vi "GUI_Single Button Pump.vi"() -> ()   [LabVIEW 2011]
uses:
  LB Status Named_typdef.ctl
  LB Statusboolarray1_typdef.ctl
  LB Statusboolarray2_typdef.ctl
  LB Statusboolarray3_typdef.ctl
  LB statusintegerarray_typdef.ctl
  LB statusfloatrarray_typdef.ctl
  EC Status Named_typdef.ctl
  EC Statusboolarray2_typdef.ctl
  EC Statusboolarray3_typdef.ctl
  EC Statusboolarray1_typdef.ctl
  EC statusintegerarray_typdef.ctl
  EC statusfloatrarray_typdef.ctl
  GPM Mode_typdef.ctl
  User Event Data Type typdef.ctl
  Error Action.ctl
  Error codes.ctl
  DecisionCluster_typdef.ctl
  MainCluster_typdef.ctl
  Chamber Selection_typdef.ctl
  timerAction_typdef.ctl
  action_typdef.ctl
  op_typdef.ctl
  Selection Action_typdef.ctl
  command_typdef.ctl
panel:
  in  "Tab Control":enum32{"Control", "Debug LB", "Debug EC"}(tab)
  in  "Pump":bool
  in  "Current State":string
  in  "Display Message":string
  in  "Errors/Warnings":i32(listbox)=1
  in  "OK":bool
  in  "GPM Mode":T1
  in  "Debug Mode?":bool
  in  "LB Status Named":T2
  in  "EC Status Named":T8
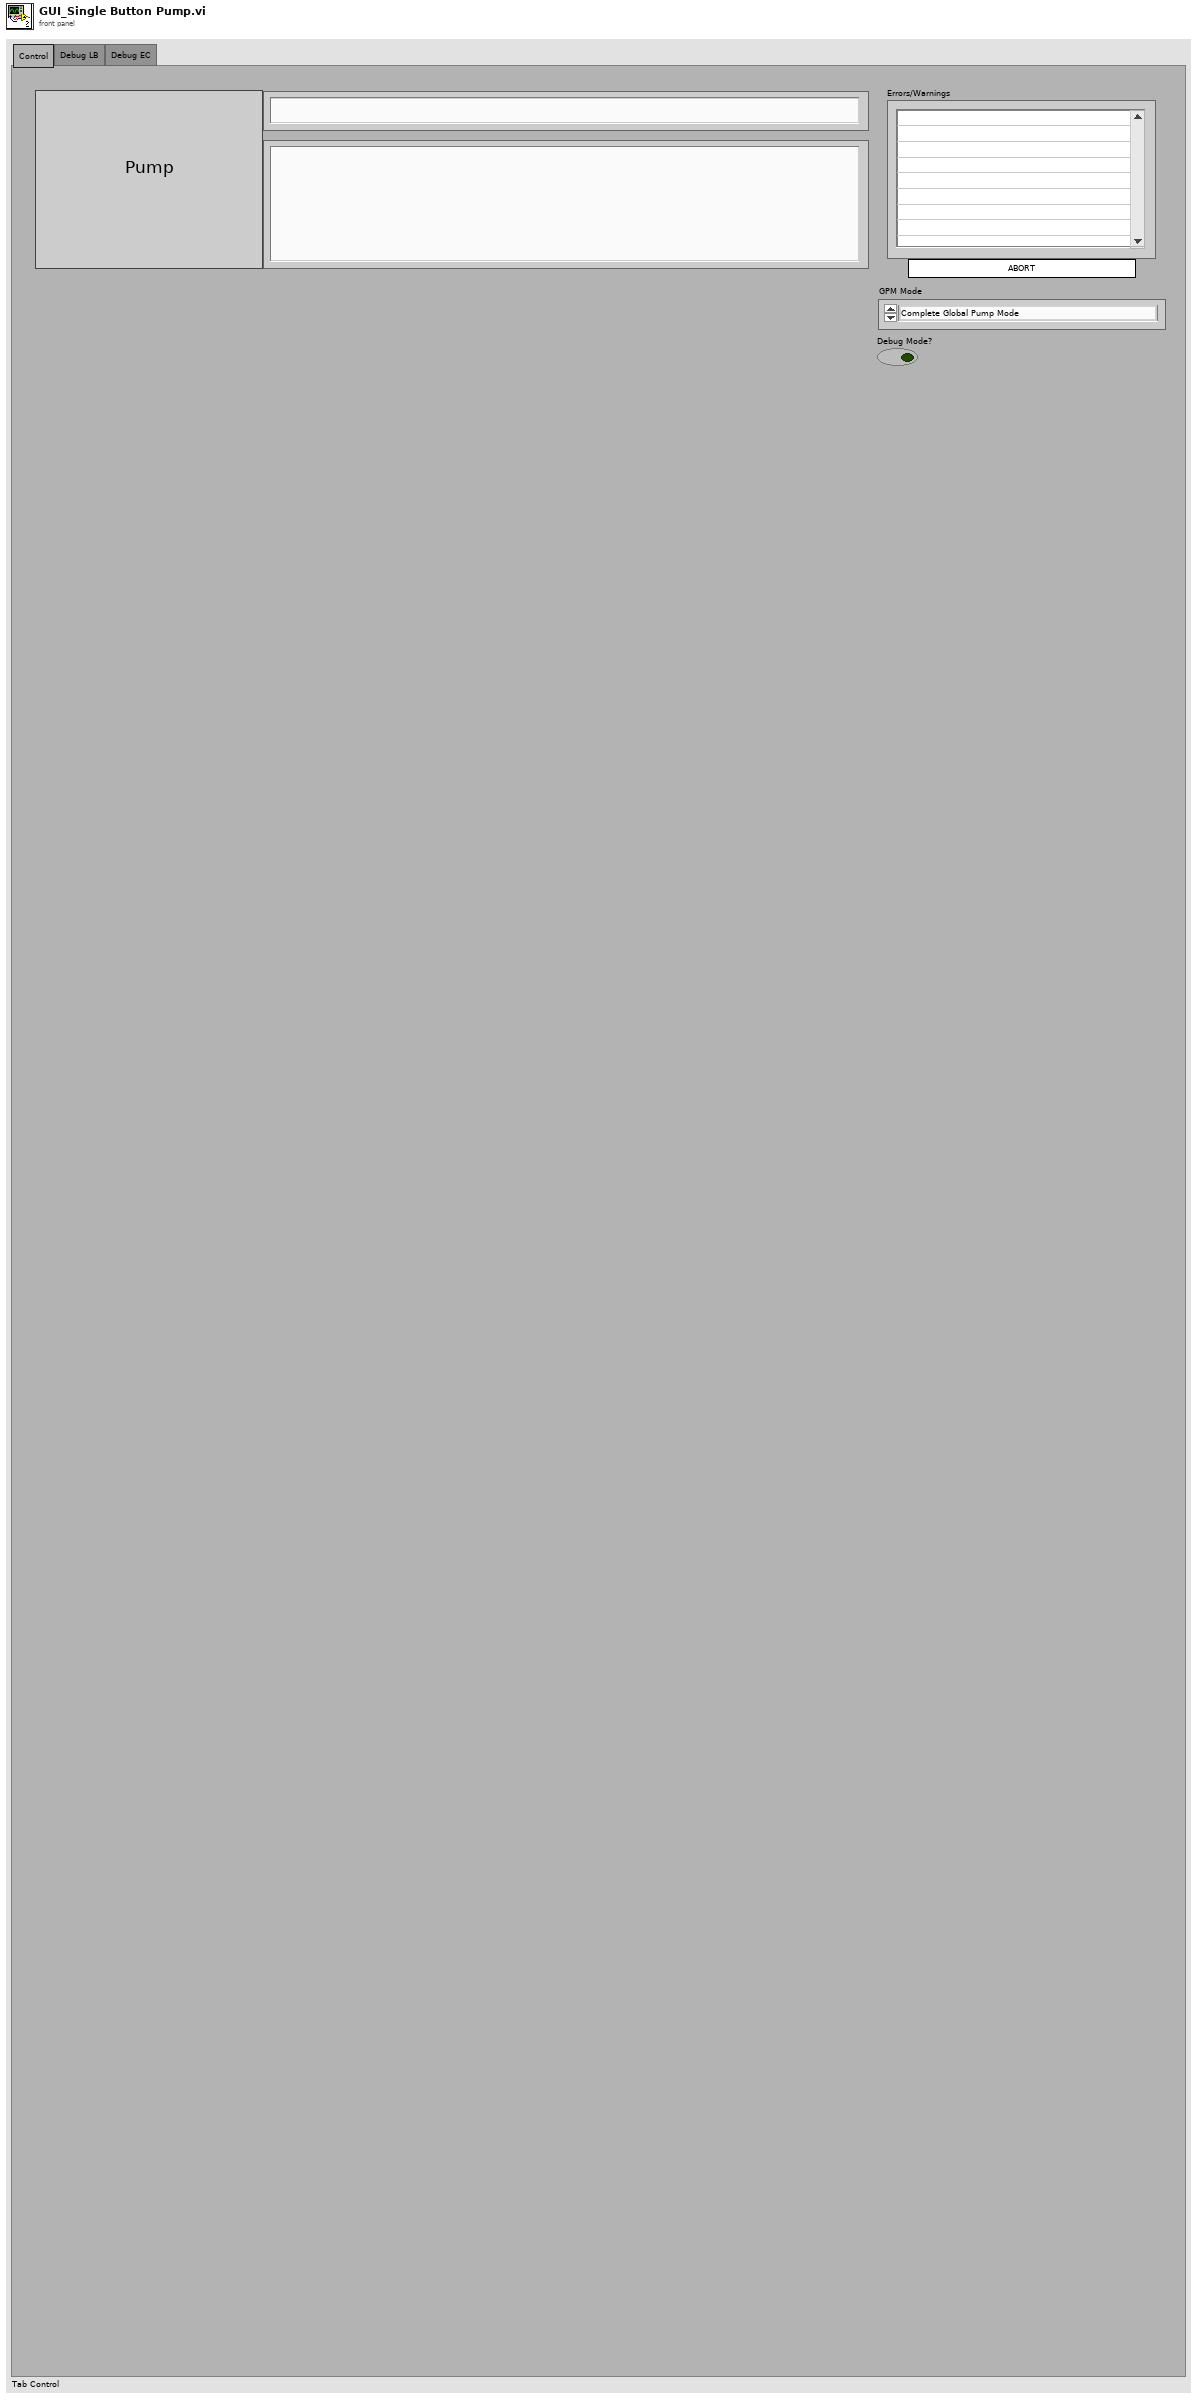
[diagram p1: front panel]
types:
  T1 = typedef "GPM Mode_typdef.ctl" = enum16{"Complete Global Pump Mode", "Selected Global Pump Mode"}
  T2 = typedef "LB Status Named_typdef.ctl" = cluster{"LB statusboolarray1":T3, "LB statusboolarray2":T4, "LB statusboolarray3":T5, "LB statusintegerarray":T6, "LB statusfloatarray":T7}
  T3 = typedef "LB Statusboolarray1_typdef.ctl" = cluster{"COMP ion gauge on feedback":bool, "COMP ion gauge degas feedback":bool, "M123 ion gauge on feedback":bool, "M123 ion gauge degas feedback":bool, "OAP ion gauge on feedback":bool, "OAP ion gauge degas feedback":bool, "Spare 1":bool, "Spare 2":bool, "Spare 3":bool, "Spare 4":bool, "Spare 5":bool, "Spare 6":bool, "ROUGHING MANIFOLD VALVE opened":bool, "ROUGHING MANIFOLD VALVE closed":bool, "BACKING MANIFOLD VALVE opened":bool, "BACKING MANIFOLD VALVE closed":bool, "ROUGHING BACKING CONNECT VALVE opened":bool, "ROUGHING BACKING CONNECT VALVE closed":bool, "COMPRESSOR ROUGHING VALVE opened":bool, "COMPRESSOR ROUGHING VALVE closed":bool, "M123 ROUGHING VALVE opened":bool, "M123 ROUGHING VALVE closed":bool, "BEAMDUMP ROUGHING VALVE opened":bool, "BEAMDUMP ROUGHING VALVE closed":bool, "OAP ROUGHING VALVE opened":bool, "OAP ROUGHING VALVE closed":bool, "GATE VALVE COMP-M123 opened":bool, "GATE VALVE COMP-M123 closed":bool, "GATE VALVE BEAM DUMP opened":bool, "GATE VALVE BEAM DUMP closed":bool, "GATE VALVE M123-OAP opened":bool, "GATE VALVE M123-OAP closed":bool, "GATE VALVE OAP-BTL opened":bool, "GATE VALVE OAP-BTL closed":bool, "COMPRESSOR VENT VALVE opened":bool, "COMPRESSOR VENT VALVE closed":bool, "M123 VENT VALVE opened":bool, "M123 VENT VALVE closed":bool, "BEAMDUMP VENT VALVE opened":bool, "BEAMDUMP VENT VALVE closed":bool, "OAP VENT VALVE opened":bool, "OAP VENT VALVE closed":bool, "COMPRESSOR Turbo Gate Valve opened ":bool, "COMPRESSOR Turbo Gate Valve closed":bool, "M123 Turbo Gate Valve opened":bool, "M123 Turbo Gate Valve closed":bool, "OAP Turbo Gate Valve opened":bool, "OAP Turbo Gate Valve closed":bool, "COMPRESSOR Turbo Backing Valve opened":bool, "COMPRESSOR Turbo Backing Valve closed":bool, "M123 Turbo Backing Valve opened":bool, "M123 Turbo Backing Valve closed":bool, "OAP Turbo Backing Valve opened":bool, "OAP Turbo Backing Valve closed":bool, "Roughing Manifold Vent Valve opened":bool, "Roughing Manifold Vent Valve closed":bool, "Spare 7":bool, "Spare 8":bool, "Spare 9":bool, "Spare 10":bool, "RP RUN opened":bool, "RP no FAULT closed":bool, "BP RUN opened":bool, "BP no FAULT closed":bool}
  T4 = typedef "LB Statusboolarray2_typdef.ctl" = cluster{"Spare 1":bool, "Spare 2":bool, "Spare 3":bool, "Spare 4":bool, "ROUGHING PUMP run":bool, "ROUGHING PUMP no fault":bool, "BACKING PUMP run":bool, "BACKING PUMP no fault":bool, "COMP TURBO fault feedback":bool, "COMP TURBO normal feedback":bool, "M123 TURBO fault feedback":bool, "M123 TURBO normal feedback":bool, "OAP TURBO fault feedback":bool, "OAP TURBO normal feedback":bool, "Spare 9":bool, "Spare 10":bool, "Spare 11":bool, "Spare 12":bool, "Spare 13":bool, "Spare 14":bool, "ROUGHING PUMP FLOW SWITCH":bool, "BACKING PUMP FLOW SWITCH":bool, "COMP TURBO FLOW SWITCH":bool, "M123 TURBO FLOW SWITCH":bool, "OAP TURBO FLOW SWITCH":bool, "Spare 15":bool, "Spare 16":bool, "Spare 17":bool, "COMP ion gauge on signal":bool, "COMP ion gauge degas signal":bool, "M123 ion gauge on signal":bool, "M123 ion gauge degas signal":bool, "OAP ion gauge on signal":bool, "OAP ion gauge degas signal":bool, "Spare 18":bool, "Spare 19":bool, "Spare 20":bool, "Spare 21":bool, "Spare 22":bool, "Spare 23":bool, "ROUGHING MANIFOLD VALVE":bool, "BACKING MANIFOLD VALVE":bool, "ROUGHING BACKING CONNECT VALVE":bool, "COMPRESSOR ROUGHING VALVE":bool, "M123 ROUGHING VALVE":bool, "BEAMDUMP ROUGHING VALVE":bool, "OAP ROUGHING VALVE":bool, "GATE VALVE COMP-M123":bool, "GATE VALVE BEAM DUMP":bool, "GATE VALVE M123-OAP":bool, "GATE VALVE OAP-BTL":bool, "COMPRESSOR VENT VALVE":bool, "M123 VENT VALVE":bool, "BEAMDUMP VENT VALVE":bool, "OAP VENT VALVE":bool, "COMPRESSOR Turbo Gate Valve":bool, "M123 Turbo Gate Valve":bool, "OAP Turbo Gate Valve":bool, "COMPRESSOR Turbo Backing Valve":bool, "M123 Turbo Backing Valve":bool, "OAP Turbo Backing Valve":bool, "Spare 24":bool, "Spare 25":bool, "Spare 26":bool}
  T5 = typedef "LB Statusboolarray3_typdef.ctl" = cluster{"Spare 1":bool, "Spare 2":bool, "Spare 3":bool, "Spare 4":bool, "ROUGHING PUMP":bool, "BACKING PUMP":bool, "Spare 5":bool, "Spare 6":bool, "Spare 7":bool, "Spare 8":bool, "Spare 9":bool, "COMP Turbo Vent Valve":bool, "M123 Turbo Vent Valve":bool, "OAP Turbo Vent Valve":bool, "Spare 10":bool, "Spare 11":bool, "Spare 12":bool, "Spare 13":bool, "COMP turbo pump run signal":bool, "M123 turbo pump run signal":bool, "OAP turbo pump run signal":bool, "Spare 14":bool, "Spare 15":bool, "Spare 16":bool, "watch dog timer - out":bool, "GATE OAP-BTL - closed out":bool, "GATE 1 – closed out":bool, "GATE 2 – closed out":bool, "GATE 3,4 – closed out":bool, "GPM LB - out":bool, "GVM LB - out":bool, "RP LB status - out":bool, "RP EC - toggle - out":bool, "Spare 17":bool, "Spare 18":bool, "Spare 19":bool, "Spare 20":bool, "Spare 21":bool, "Spare 22":bool, "Spare 23":bool}
  T6 = typedef "LB statusintegerarray_typdef.ctl" = cluster{"COMP vacuum status word convectron ATM":i32, "M123 vacuum status word convectron ATM":i32, "OAP vacuum status word convectron ATM":i32, "HPBD vacuum status word convectron ATM":i32, "Spare 1":i32, "Spare 2":i32, "roughing pump vacuum status word convectron":i32, "backing pump vacuum status word convectron":i32, "roughing manifold vacuum status word convectron":i32, "backing manifold vacuum status word convectron":i32, "COMP Convectron vacuum status word convectron":i32, "M123 Convectron vacuum status word convectron":i32, "OAP Convectron vacuum status word convectron":i32, "Spare 3":i32, "Spare 4":i32, "COMP status word turbo pump":i32, "M123 status word turbo pump":i32, "OAP status word turbo pump":i32, "Spare 5":i32, "Spare 6":i32, "Spare 7":i32, "Spare 8":i32, "Spare 9":i32, "Spare 10":i32, "COMP CONVECTRON consloidate":i32, "Spare 11":i32, "Spare 12":i32, "Spare 13":i32, "M123 CONVECTRON consloidate":i32, "Spare 14":i32, "Spare 15":i32, "Spare 16":i32, "OAP CONVECTRON consloidate":i32, "Spare 17":i32, "Spare 18":i32, "Spare 19":i32, "HPBD CONVECTRON consloidate":i32, "Spare 20":i32, "Spare 21":i32, "Spare 22":i32, "Spare 23":i32, "Spare 24":i32, "Spare 25":i32, "Spare 26":i32, "Spare 27":i32, "Spare 28":i32, "Spare 29":i32, "Spare 30":i32}
  T7 = typedef "LB statusfloatrarray_typdef.ctl" = cluster{"COMP READING ION GAUGE":dbl, "M123 READING ION GAUGE":dbl, "OAP READING ION GAUGE":dbl, "Spare 1":i32, "Spare 2":i32, "Spare 3":i32, "Spare 4":i32, "Spare 5":i32, "roughing pump CONVECTRON GAUGE":dbl, "backing pump CONVECTRON GAUGE":dbl, "roughing manifold CONVECTRON GAUGE":dbl, "backing manifold CONVECTRON GAUGE":dbl, "COMP Convectron CONVECTRON GAUGE":dbl, "M123 Convectron CONVECTRON GAUGE":dbl, "OAP Convectron CONVECTRON GAUGE":dbl, "Spare 6":i32, "Spare 7":i32, "Spare 8":i32, "Spare 9":i32, "Spare 10":i32, "Spare 11":i32, "Spare 12":i32, "Spare 13":i32, "Spare 14":i32}
  T8 = typedef "EC Status Named_typdef.ctl" = cluster{"EC statusboolarray2":T9, "EC statusboolarray3":T10, "EC statusboolarray1":T11, "EC statusintegerarray":T12, "EC statusfloatarray":T13}
  T9 = typedef "EC Statusboolarray2_typdef.ctl" = cluster{"Spare 1":bool, "Spare 2":bool, "Spare 3":bool, "Spare 4":bool, "ROUGHING PUMP run opened":bool, "ROUGHING PUMP no fault closed":bool, "BACKING PUMP run opened":bool, "BACKING PUMP no fault closed":bool, "BTL TURBO turbo fault feedback":bool, "BTL TURBO turbo normal feedback":bool, "TARGET 1 TURBO turbo fault feedback":bool, "TARGET 1 TURBO turbo normal feedback":bool, "TARGET 2 TURBO turbo fault feedback":bool, "TARGET 2 TURBO turbo normal feedback":bool, "BTL2 TURBO turbo fault feedback":bool, "BTL2 TURBO turbo normal feedback":bool, "HPD TURBO turbo fault feedback":bool, "HPD TURBO turbo normal feedback":bool, "Spare 5":bool, "Spare 6":bool, "ROUGHING PUMP FLOW SWITCH":bool, "BACKING PUMP FLOW SWITCH":bool, "BTL TURBO FLOW SWITCH":bool, "TARGET 1 TURBO FLOW SWITCH":bool, "TARGET 2 TURBO FLOW SWITCH":bool, "BTL2 TURBO FLOW SWITCH":bool, "HPD TURBO FLOW SWITCH":bool, "Spare 7":bool, "BTL ion gauge on signal":bool, "BTL ion gauge degas signal":bool, "TARGET ion gauge on signal":bool, "TARGET ion gauge degas signal":bool, "BTL2 ion gauge on signal":bool, "BTL2 ion gauge degas signal":bool, "HPD ion gauge on signal":bool, "HPD ion gauge degas signal":bool, "Spare 8":bool, "Spare 9":bool, "Spare 10":bool, "Spare 11":bool, "ROUGHING MANIFOLD VALVE":bool, "BACKING MANIFOLD VALVE":bool, "ROUGHING BACKING CONNECT VALVE":bool, "BTL ROUGHING VALVE":bool, "BTL VENT VALVE":bool, "BTL Turbo Gate Valve":bool, "BTL Turbo Backing Valve":bool, "Roughing Manifold VV":bool, "Backing Manifold VV":bool, "TARGET ROUGHING VALVE":bool, "BTL2 ROUGHING VALVE":bool, "HPD ROUGHING VALVE":bool, "GV BTL-TARGET":bool, "GV TARGET-BTL2":bool, "GV BTL2-HPD":bool, "TARGET VENT VALVE":bool, "BTL2 VENT VALVE":bool, "HPD VENT VALVE":bool, "TARGET  Turbo Gate Valve 1":bool, "TARGET  Turbo Gate Valve 2":bool, "BTL2 Turbo Gate Valve":bool, "HPD  Turbo Gate Valve":bool, "TARGET Turbo Backing Valve 1":bool, "TARGET Turbo Backing Valve 2":bool}
  T10 = typedef "EC Statusboolarray3_typdef.ctl" = cluster{"BTL2 Turbo Backing Valve":bool, "HPD Turbo Backing Valve":bool, "Spare 1":bool, "Spare 2":bool, "Spare 3":bool, "Spare 4":bool, "Spare 5":bool, "Spare 6":bool, "Spare 7":bool, "Spare 8":bool, "Spare 9":bool, "BTL Turbo Vent Valve":bool, "TARGET1 Turbo Vent Valve":bool, "TARGET2 Turbo Vent Valve":bool, "BTL2 Turbo Vent Valve":bool, "HPD Turbo Vent Valve":bool, "Spare 10":bool, "Spare 11":bool, "BTL turbo pump run signal":bool, "TARGET1 turbo pump run signal":bool, "TARGET2 turbo pump run signal":bool, "BTL2 turbo pump run signal":bool, "HPD turbo pump run signal":bool, "Spare 12":bool, "watch dog timer - out":bool, "BTL vented – out":bool, "BTL medvac – out":bool, "BTL hivac – out":bool, "GPM EC - out":bool, "GVM EC - out":bool, "RP EC status - out":bool, "RP LB toggle - out":bool, "GATE ALL - closed out":bool, "Spare 13":bool, "Spare 14":bool, "Spare 15":bool, "Spare 16":bool, "Spare 17":bool, "Spare 18":bool, "Spare 19":bool, "Spare 20":bool, "Spare 21":bool, "Spare 22":bool, "Spare 23":bool, "Spare 24":bool, "Spare 25":bool, "Spare 26":bool, "Spare 27":bool}
  T11 = typedef "EC Statusboolarray1_typdef.ctl" = cluster{"BTL ion gauge on feedback":bool, "BTL ion gauge degas feedback":bool, "TARGET ion gauge on feedback":bool, "TARGET ion gauge degas feedback":bool, "BTL2 ion gauge on feedback":bool, "BTL2 ion gauge degas feedback":bool, "HPD ion gauge on feedback":bool, "HPD ion gauge degas feedback":bool, "Spare 1":bool, "Spare 2":bool, "Spare 3":bool, "Spare 4":bool, "ROUGHING MANIFOLD VALVE opened":bool, "ROUGHING MANIFOLD VALVE closed":bool, "BACKING MANIFOLD VALVE opened":bool, "BACKING MANIFOLD VALVE closed":bool, "ROUGHING BACKING CONNECT VALVE opened":bool, "ROUGHING BACKING CONNECT VALVE closed":bool, "BTL ROUGHING VALVE opened":bool, "BTL ROUGHING VALVE closed":bool, "BTL VENT VALVE opened":bool, "BTL VENT VALVE closed":bool, "BTL Turbo Gate Valve opened":bool, "BTL Turbo Gate Valve closed":bool, "BTL Turbo Backing Valve opened":bool, "BTL Turbo Backing Valve closed":bool, "Roughing Manifold VV opened":bool, "Roughing Manifold VV closed":bool, "Backing Manifold VV opened":bool, "Backing Manifold VV closed":bool, "TARGET ROUGHING VALVE opened":bool, "TARGET ROUGHING VALVE closed":bool, "BTL2 ROUGHING VALVE opened":bool, "BTL2 ROUGHING VALVE closed":bool, "HPD ROUGHING VALVE opened":bool, "HPD ROUGHING VALVE closed":bool, "GV BTL-TARGET opened":bool, "GV BTL-TARGET closed":bool, "GV TARGET-BTL2 opened":bool, "GV TARGET-BTL2 closed":bool, "GV BTL2-HPD opened":bool, "GV BTL2-HPD closed":bool, "TARGET VENT VALVE opened":bool, "TARGET VENT VALVE closed":bool, "BTL2 VENT VALVE opened":bool, "BTL2 VENT VALVE closed":bool, "HPD VENT VALVE opened":bool, "HPD VENT VALVE closed":bool, "TARGET  Turbo Gate Valve 1 opened":bool, "TARGET  Turbo Gate Valve 1 closed":bool, "TARGET  Turbo Gate Valve 2 opened":bool, "TARGET  Turbo Gate Valve 2 closed":bool, "BTL2 Turbo Gate Valve opened":bool, "BTL2 Turbo Gate Valve closed":bool, "HPD  Turbo Gate Valve opened":bool, "HPD  Turbo Gate Valve closed":bool, "TARGET Turbo Backing Valve 1 opened":bool, "TARGET Turbo Backing Valve 1 closed":bool, "TARGET Turbo Backing Valve 2 opened":bool, "TARGET Turbo Backing Valve 2 closed":bool, "BTL2 Turbo Backing Valve opened":bool, "BTL2 Turbo Backing Valve closed":bool, "HPD Turbo Backing Valve opened":bool, "HPD Turbo Backing Valve closed":bool}
  T12 = typedef "EC statusintegerarray_typdef.ctl" = cluster{"BTL vacuum status word convectron ATM":i32, "TARGET vacuum status word convectron ATM 2":i32, "BTL2 vacuum status word convectron ATM 3":i32, "HPD vacuum status word convectron ATM 4":i32, "Spare 1":i32, "Spare 2":i32, "roughing pump vacuum status word convectron":i32, "backing pump vacuum status word convectron":i32, "roughing manifold vacuum status word convectron":i32, "backing manifold vacuum status word convectron":i32, "BTL Convectron vacuum status word convectron":i32, "TARGET1 Convectron vacuum status word convectron":i32, "TARGET2 Convectron vacuum status word convectron":i32, "BTL2 Convectron vacuum status word convectron":i32, "HPD Convectron vacuum status word convectron":i32, "BTL status word turbo pump":i32, "TARGET1 status word turbo pump":i32, "TARGET2 status word turbo pump":i32, "BTL2 status word turbo pump??":i32, "HPD status word turbo pump":i32, "Spare 3":i32, "Spare 4":i32, "Spare 5":i32, "Spare 6":i32, "BTL CONVECTRON Consolidate":i32, "Spare 7":i32, "Spare 8":i32, "Spare 9":i32, "TARGET Consolidate":i32, "Spare 10":i32, "Spare 11":i32, "Spare 12":i32, "BTL2 Consolidate":i32, "Spare 13":i32, "Spare 14":i32, "Spare 15":i32, "HPD Consolidate":i32, "Spare 16":i32, "Spare 17":i32, "Spare 18":i32, "Spare 19":i32, "Spare 20":i32, "Spare 21":i32, "Spare 22":i32, "Spare 23":i32, "Spare 24":i32, "Spare 25":i32, "Spare 26":i32}
  T13 = typedef "EC statusfloatrarray_typdef.ctl" = cluster{"BTL READING ION GAUGE":dbl, "TARGET READING ION GAUGE":dbl, "BTL2 READING ION GAUGE":dbl, "HPD READING ION GAUGE":dbl, "Spare 1":dbl, "Spare 2":dbl, "Spare 3":dbl, "Spare 4":dbl, "roughing pump READING CONVECTRON GAUGE":dbl, "backing pump READING CONVECTRON GAUGE":dbl, "roughing manifold READING CONVECTRON GAUGE":dbl, "backing manifold READING CONVECTRON GAUGE":dbl, "BTL Convectron READING CONVECTRON GAUGE":dbl, "TARGET1 READING CONVECTRON GAUGE":dbl, "TARGET2 READING CONVECTRON GAUGE":dbl, "BTL2 READING CONVECTRON GAUGE":dbl, "HPD READING CONVECTRON GAUGE":dbl, "Spare 5":dbl, "Spare 6":dbl, "Spare 7":dbl, "Spare 8":dbl, "Spare 9":dbl, "Spare 10":dbl, "Spare 11":dbl}
  T14 = typedef "DecisionCluster_typdef.ctl" = cluster{"vi path":path, "Message":string}
  T15 = typedef "User Event Data Type typdef.ctl" = cluster{"Error Action":T16, "Error Codes":T17, "Status Array":string[]}
  T16 = typedef "Error Action.ctl" = enum16{"Add", "Remove", "Read All"}
  T17 = typedef "Error codes.ctl" = enum16{"001-GPM and GVM conditions", "002-Turbo gate valve status", "003-Chamber Gate Valve Status", "004-Check Chamber Pressures", "005-Check GPM Handshake", "006-Roughing Pump Status", "007-Backing Pump Status", "008-Backing valve status", "009-Roughing Manifold Pressure Status", "010-Roughing Valve Status", "011-Roughing Pump Status", "012-Turbo Backing Valve Status", "013-MID-VAC Status", "999-No Event"}
  T18 = enum8{"Enabled", "Disabled", "Disabled and Grayed Out"}
  T19 = enum32{"invalid app kind", "Development System", "Run Time System", "Student Edition", "Embedded LabVIEW", "Evaluation", "Custom"}
  T20 = typedef "MainCluster_typdef.ctl" = cluster{"Isolate HPBD":bool, "Core":cluster{"Current VI Reference":refnum<vi>, "Close Panel on Exit?":bool}, "Status Display Array":string[], "Connection URLs":cluster{"Source_URL EC":string, "Target_URL EC":string, "Source_URL LB":string, "Target_URL LB":string}, "EC Status":cluster{"bits 2":bool[], "bits 2":bool[], "bits 2":bool[], i32[], "FLOAT NUMBERS 2":sgl[]}, "EC Status Named":T8, "TCPConnection":cluster{"Status TCP Connection EC":refnum<k5>, "Command TCP Connection EC":refnum<k5>, "Status TCP Connection LB":refnum<k5>, "Command TCP Connection LB":refnum<k5>}, "EC Command Cluster":cluster{"boolarray1":cluster{bool, bool, bool, bool, bool, bool, bool, bool, bool, bool, bool, bool, bool, bool, bool, bool}, "boolarray2":cluster{bool, bool, bool, bool, bool, bool, bool, bool, bool, bool, bool, bool, bool, bool, bool, bool}, "boolarray3":cluster{bool, bool, bool, bool, bool, bool, bool, bool, bool, bool, bool, bool, bool, bool, bool, bool}, "boolarray4":cluster{bool, bool, bool, bool, bool, bool, bool, bool, bool, bool, bool, bool, bool, bool, bool, bool}}, "EC Command Named":cluster{"EC Command array 1":cluster{"ROUGHING MANIFOLD VALVE":bool, "BACKING MANIFOLD VALVE":bool, "ROUGHING BACKING CONNECT VALVE":bool, "BTL ROUGHING VALVE":bool, "BTL VENT VALVE":bool, "BTL Turbo Gate Valve":bool, "BTL Turbo Backing Valve":bool, "Roughing Manifold VV":bool, "Backing Manifold VV":bool, "TARGET ROUGHING VALVE":bool, "BTL2 ROUGHING VALVE":bool, "HPD ROUGHING VALVE":bool, "GV BTL-TARGET":bool, "GV TARGET-BTL2":bool, "GV BTL2-HPD":bool, "TARGET VENT VALVE":bool}, " EC Command array 2":cluster{"BTL2 VENT VALVE":bool, "HPD VENT VALVE":bool, "TARGET  Turbo Gate Valve 1":bool, "TARGET  Turbo Gate Valve 2":bool, "BTL2 Turbo Gate Valve":bool, "HPD  Turbo Gate Valve":bool, "TARGET Turbo Backing Valve 1":bool, "TARGET Turbo Backing Valve 2":bool, "BTL2 Turbo Backing Valve":bool, "HPD Turbo Backing Valve":bool, "Spare 1":bool, "Spare 2":bool, "ROUGHING PUMP":bool, "BACKING PUMP":bool, "Spare 3":bool, "Spare 4":bool}, "EC Command array 3":cluster{"Spare 1":bool, "Spare 2":bool, "Spare 3":bool, "BTL Turbo Vent Valve":bool, "TARGET1 Turbo Vent Valve":bool, "TARGET2 Turbo Vent Valve":bool, "BTL2 Turbo Vent Valve":bool, "HPD Turbo Vent Valve":bool, "Spare 4":bool, "Spare 5":bool, "GPM":bool, "GVM":bool, "Spare 6":bool, "BTL turbo pump":bool, "TARGET1 turbo pump":bool, "TARGET2 turbo pump":bool}, "EC Command array 4":cluster{"BLT turbo pump":bool, "HPD turbo pump":bool, "Spare 1":bool, "BTL ION GAUGE ion gauge":bool, "BTL ION GAUGE  ion gauge degas":bool, "TARGET ion gauge":bool, "TARGET ion gauge degas":bool, "BTL2 ion gauge":bool, "BTL2 ion gauge degas":bool, "HPD ion gauge":bool, "HPD ion gauge degas":bool, "Spare 2":bool, "Spare 3":bool, "Spare 4":bool, "Spare 5":bool, "Spare 6":bool}}, "LB Status Named":T2, "LB Status":cluster{"bits 2":bool[], "bits 2":bool[], "bits 2":bool[], i32[], "FLOAT NUMBERS 2":sgl[]}, "LB Command Cluster":cluster{"boolarray1":cluster{bool, bool, bool, bool, bool, bool, bool, bool, bool, bool, bool, bool, bool, bool, bool, bool}, "boolarray2":cluster{bool, bool, bool, bool, bool, bool, bool, bool, bool, bool, bool, bool, bool, bool, bool, bool}, "boolarray3":cluster{bool, bool, bool, bool, bool, bool, bool, bool, bool, bool, bool, bool, bool, bool, bool, bool}, "boolarray4":cluster{bool, bool, bool, bool, bool, bool, bool, bool, bool, bool, bool, bool, bool, bool, bool, bool}}, "LB Command Named":cluster{"LB commandarray1":cluster{"ROUGHING MANIFOLD VALVE":bool, "BACKING MANIFOLD VALVE":bool, "ROUGHING BACKING CONNECT VALVE":bool, "COMPRESSOR ROUGHING VALVE":bool, "M123 ROUGHING VALVE":bool, "BEAMDUMP ROUGHING VALVE":bool, "OAP ROUGHING VALVE":bool, "GATE VALVE COMP-M123":bool, "GATE VALVE BEAM DUMP":bool, "GATE VALVE M123-OAP":bool, "GATE VALVE OAP-BTL":bool, "COMPRESSOR VENT VALVE":bool, "M123 VENT VALVE":bool, "BEAMDUMP VENT VALVE":bool, "OAP VENT VALVE":bool, "COMPRESSOR Turbo Gate Valve":bool}, "LB commandarray2":cluster{"M123 Turbo Gate Valve":bool, "OAP Turbo Gate Valve":bool, "COMPRESSOR Turbo Backing Valve":bool, "M123 Turbo Backing Valve":bool, "OAP Turbo Backing Valve":bool, "Roughing Manifold Vent Valve":bool, "Backing Manifold Vent Valve":bool, "Spare 1":bool, "Spare 2":bool, "Spare 3":bool, "Spare 4":bool, "Spare 5":bool, "ROUGHING PUMP":bool, "BACKING PUMP":bool, "Spare 6":bool, "Spare 7":bool}, "LB commandarray3":cluster{"Spare 1":bool, "Spare 2":bool, "Spare 3":bool, "COMP Turbo Vent Valve":bool, "M123 Turbo Vent Valve":bool, "OAP Turbo Vent Valve":bool, "Spare 4":bool, "Spare 5":bool, "Spare 6":bool, "Spare 7":bool, "GPM":bool, "GVM":bool, "Spare 8":bool, "COMP turbo pump":bool, "M123 turbo pump":bool, "OAP turbo pump":bool}, "LB commandarray4":cluster{"Spare 1":bool, "Spare 2":bool, "Spare 3":bool, "COMP ION GAUGE":bool, "COMP ION GAUGE degas":bool, "M123 ION GAUGE":bool, "M123 ION GAUGE degas":bool, "OAP ION GAUGE":bool, "OAP ION GAUGE degas":bool, "Spare 4":bool, "Spare 5":bool, "Spare 6":bool, "Spare 7":bool, "Spare 8":bool, "Spare 9":bool, "Spare 10":bool}}, "VI Refnum":refnum<vi>, "Chamber Selection":T21, "GPM Mode":T1, "Debug Mode?":bool, "State Sanity Check Array":bool[], "Critical Failures":cluster{"GPM Exit?":bool}, "Comm Ready?":bool, "Status Reconnect Attempt":dbl}
  T21 = typedef "Chamber Selection_typdef.ctl" = cluster{"COMP":bool, "M123":bool, "HPBD":bool, "OAP":bool, "BTL":bool, "TARGET":bool, "BTL2":bool, "HPD":bool}
  T22 = typedef "timerAction_typdef.ctl" = enum16{"Idle", "Start Timer", "Timer Running"}
  T23 = enum32{"Invalid", "Standard", "Closed", "Hidden", "Minimized", "Maximized"}
  T24 = typedef "op_typdef.ctl" = enum16{"Idle", "Continue to Wait", "Exit", "Ignore and Continue"}
  T25 = typedef "Selection Action_typdef.ctl" = enum16{"No Action", "Check Chamber Pressure", "Check Turbo Gate Valves", "Open Turbo Backing Valves", "Check Turbo Backing Valves", "Check MID-VAC on Chambers", "Start Turbo Pumps", "Check Turbo Normal Operation", "Check Chamber Pressures", "Roughing Valve Selection"}
  T26 = cluster{"bits 2":bool[], "bits 2":bool[], "bits 2":bool[], i32[], "FLOAT NUMBERS 2":sgl[]}
  T27 = cluster{"bits 2[0]":bool, "bits 2[1]":bool, "bits 2[2]":bool, "bits 2[3]":bool, "bits 2[4]":bool, "bits 2[5]":bool, "bits 2[6]":bool, "bits 2[7]":bool, "bits 2[8]":bool, "bits 2[9]":bool, "bits 2[10]":bool, "bits 2[11]":bool, "bits 2[12]":bool, "bits 2[13]":bool, "bits 2[14]":bool, "bits 2[15]":bool, "bits 2[16]":bool, "bits 2[17]":bool, "bits 2[18]":bool, "bits 2[19]":bool, "bits 2[20]":bool, "bits 2[21]":bool, "bits 2[22]":bool, "bits 2[23]":bool, "bits 2[24]":bool, "bits 2[25]":bool, "bits 2[26]":bool, "bits 2[27]":bool, "bits 2[28]":bool, "bits 2[29]":bool, "bits 2[30]":bool, "bits 2[31]":bool, "bits 2[32]":bool, "bits 2[33]":bool, "bits 2[34]":bool, "bits 2[35]":bool, "bits 2[36]":bool, "bits 2[37]":bool, "bits 2[38]":bool, "bits 2[39]":bool, "bits 2[40]":bool, "bits 2[41]":bool, "bits 2[42]":bool, "bits 2[43]":bool, "bits 2[44]":bool, "bits 2[45]":bool, "bits 2[46]":bool, "bits 2[47]":bool, "bits 2[48]":bool, "bits 2[49]":bool, "bits 2[50]":bool, "bits 2[51]":bool, "bits 2[52]":bool, "bits 2[53]":bool, "bits 2[54]":bool, "bits 2[55]":bool, "bits 2[56]":bool, "bits 2[57]":bool, "bits 2[58]":bool, "bits 2[59]":bool, "bits 2[60]":bool, "bits 2[61]":bool, "bits 2[62]":bool, "bits 2[63]":bool}
  T28 = cluster{"FLOAT NUMBERS 2[0]":sgl, "FLOAT NUMBERS 2[1]":sgl, "FLOAT NUMBERS 2[2]":sgl, "FLOAT NUMBERS 2[3]":sgl, "FLOAT NUMBERS 2[4]":sgl, "FLOAT NUMBERS 2[5]":sgl, "FLOAT NUMBERS 2[6]":sgl, "FLOAT NUMBERS 2[7]":sgl, "FLOAT NUMBERS 2[8]":sgl, "FLOAT NUMBERS 2[9]":sgl, "FLOAT NUMBERS 2[10]":sgl, "FLOAT NUMBERS 2[11]":sgl, "FLOAT NUMBERS 2[12]":sgl, "FLOAT NUMBERS 2[13]":sgl, "FLOAT NUMBERS 2[14]":sgl, "FLOAT NUMBERS 2[15]":sgl, "FLOAT NUMBERS 2[16]":sgl, "FLOAT NUMBERS 2[17]":sgl, "FLOAT NUMBERS 2[18]":sgl, "FLOAT NUMBERS 2[19]":sgl, "FLOAT NUMBERS 2[20]":sgl, "FLOAT NUMBERS 2[21]":sgl, "FLOAT NUMBERS 2[22]":sgl, "FLOAT NUMBERS 2[23]":sgl}
  T29 = cluster{"bits 2[0]":bool, "bits 2[1]":bool, "bits 2[2]":bool, "bits 2[3]":bool, "bits 2[4]":bool, "bits 2[5]":bool, "bits 2[6]":bool, "bits 2[7]":bool, "bits 2[8]":bool, "bits 2[9]":bool, "bits 2[10]":bool, "bits 2[11]":bool, "bits 2[12]":bool, "bits 2[13]":bool, "bits 2[14]":bool, "bits 2[15]":bool, "bits 2[16]":bool, "bits 2[17]":bool, "bits 2[18]":bool, "bits 2[19]":bool, "bits 2[20]":bool, "bits 2[21]":bool, "bits 2[22]":bool, "bits 2[23]":bool, "bits 2[24]":bool, "bits 2[25]":bool, "bits 2[26]":bool, "bits 2[27]":bool, "bits 2[28]":bool, "bits 2[29]":bool, "bits 2[30]":bool, "bits 2[31]":bool, "bits 2[32]":bool, "bits 2[33]":bool, "bits 2[34]":bool, "bits 2[35]":bool, "bits 2[36]":bool, "bits 2[37]":bool, "bits 2[38]":bool, "bits 2[39]":bool, "bits 2[40]":bool, "bits 2[41]":bool, "bits 2[42]":bool, "bits 2[43]":bool, "bits 2[44]":bool, "bits 2[45]":bool, "bits 2[46]":bool, "bits 2[47]":bool}
  T30 = cluster{"[0]":i32, "[1]":i32, "[2]":i32, "[3]":i32, "[4]":i32, "[5]":i32, "[6]":i32, "[7]":i32, "[8]":i32, "[9]":i32, "[10]":i32, "[11]":i32, "[12]":i32, "[13]":i32, "[14]":i32, "[15]":i32, "[16]":i32, "[17]":i32, "[18]":i32, "[19]":i32, "[20]":i32, "[21]":i32, "[22]":i32, "[23]":i32, "[24]":i32, "[25]":i32, "[26]":i32, "[27]":i32, "[28]":i32, "[29]":i32, "[30]":i32, "[31]":i32, "[32]":i32, "[33]":i32, "[34]":i32, "[35]":i32, "[36]":i32, "[37]":i32, "[38]":i32, "[39]":i32, "[40]":i32, "[41]":i32, "[42]":i32, "[43]":i32, "[44]":i32, "[45]":i32, "[46]":i32, "[47]":i32}
  T31 = cluster{"bits 2[0]":bool, "bits 2[1]":bool, "bits 2[2]":bool, "bits 2[3]":bool, "bits 2[4]":bool, "bits 2[5]":bool, "bits 2[6]":bool, "bits 2[7]":bool, "bits 2[8]":bool, "bits 2[9]":bool, "bits 2[10]":bool, "bits 2[11]":bool, "bits 2[12]":bool, "bits 2[13]":bool, "bits 2[14]":bool, "bits 2[15]":bool, "bits 2[16]":bool, "bits 2[17]":bool, "bits 2[18]":bool, "bits 2[19]":bool, "bits 2[20]":bool, "bits 2[21]":bool, "bits 2[22]":bool, "bits 2[23]":bool, "bits 2[24]":bool, "bits 2[25]":bool, "bits 2[26]":bool, "bits 2[27]":bool, "bits 2[28]":bool, "bits 2[29]":bool, "bits 2[30]":bool, "bits 2[31]":bool, "bits 2[32]":bool, "bits 2[33]":bool, "bits 2[34]":bool, "bits 2[35]":bool, "bits 2[36]":bool, "bits 2[37]":bool, "bits 2[38]":bool, "bits 2[39]":bool}
  T32 = typedef "action_typdef.ctl" = enum16{"No Action", "Is EC GPM Mode ON?", "Is EC GPM Mode Off?", "Is EC GVM Mode ON?", "Is EC GVM Off?", "Is  EC GPM or GVM Mode ON?", "Is LB GPM Mode ON?", "Is LB GPM Mode Off?", "Is LB GVM Mode ON?", "Is LB GVM Mode Off?", "Is  LB GPM or GVM Mode ON?", "Is M123 Turbo Gate Valve Opened? ", "Is M123 Turbo Gate Valve Closed?", "Is OAP Turbo Gate Valve Opened?", "Is OAP Turbo Gate Valve Closed?", "Is BTLTurbo Gate Valve Opened?", "Is BTL Turbo Gate Valve Closed?", "Is TARGET Turbo Gate Valve 1Opened?", "Is TARGET1 Turbo Gate Valve Closed?", "Is TARGET Turbo Gate Valve 2 Opened?", "Is TAREGT2 Turbo Gate Valve Closed?", "Is BTL2 Turbo Gate Valve Opened?", "Is BTL2 Turbo Gate Valve Closed?", "Is HPD Turbo Gate Valve Opened?", "Is HPD Turbo Gate Valve Closed?", "Is COMP to M123 gate Valve Opened?", "Is COMP to M123 Valve Closed?", "Is HPBD Gate Valve Opened?", "Is HPBD Gate Valve Closed?", "Is M123 to OAP gate valve opened?", "Is M123 to OAP gate valve closed?", "Is OAP to BLT gate valve opened?", "Is OAP to BTL Gate Valve Closed?", "Is BLT to TARGET gate valve opened?", "Is BTL to TARGET Gate Valve Closed?", "Is TARGET to BLT2 gate valve opened?", "Is TARGET to BTL2 Gate Valve Closed?", "Is BLT2 to HPD gate valve opened?", "Is BTL2 to HPD Gate Valve Closed?", "Is COMP at Atmospheric Pressure?", "Is M123 at Atmospheric Pressure?", "Is BeamDump at Atmospheric Pressure?", "Is OAP at Atmospheric Pressure?", "Is BLT at Atmospheric Pressure", "Is TARGET at Atmospheric Pressure?", "Is BLT2 at Atmospheric Pressure?", "Is HPD at Atmospheric Pressure?", "Is the EC Roughing Pump ON?", "Is the EC Roughing Pump OFF?", "Does the EC Roughing Pump have a fault?", "Is the LB Roughing Pump ON?", "Is the LB Roughing Pump Off?", "Does the LB Roughing Pump have a fault?", "Is the EC Backing Pump ON?", "Is the EC Backing Pump OFF?", "Is the LB Backing Pump ON?", "Is the LB Backing Pump OFF?", "Does the EC Backing Pump have a fault?", "Does the LB Backing Pump have a fault?", "Is the EC Backing Pipe at Atmospheric Pressure", "Is the LB Backing Pipe at Atmospheric Pressure", "Is the EC Backing Manifold at Atmospheric Pressure", "s the LB Backing Manifold at Atmospheric Pressure?", "Is the EC Roughing Pipe at Atmospheric Pressure", "Is the LB Roughing Pipe at Atmospheric Pressure?", "Is the EC Roughing Manifold at Atmospheric Pressure", "Is the LB Roughing Manifold at Atmospheric Pressure", "Is LB Backing Manifold Valve Opened?", "Is EC Backing Manifold Valve Opened?", "Is LB Roughing Manifold Valve Opened?", "Is EC Roughing Manifold Valve Opened?", "Is COMP Roughing Valve Opened?", "Is M123 Roughing Valve Opened?", "Is M123 Roughing Valve Closed?", "Is OAP Roughing Valve Opened?", "Is OAP Roughing Valve Closed?", "Is HPBD Roughing Valve Opened?", "Is HPBD Roughing Valve Closed?", "Is BTL Roughing Valve Opened?", "Is BTL Roughing Valve Closed?", "Is TARGET Roughing Valve Opened?", "Is TARGET Roughing Valve Closed?", "Is BTL2 Roughing Valve Opened?", "Is BTL2 Roughing Valve Closed?", "Is HPD Roughing Valve Opened?", "Is HPD Roughing Valve Closed?", "Is COMP Turbo Backing Valve Opened?", "Is M123 Turbo Backing Valve Opened", "Is HPBD Turbo Backing Valve Opened?", "Is OAP Turbo Backing Valve Opened?", "Is BTL Turbo Backing Valve Opened?", "Is TARGET1 Turbo Backing Valve Opened?", "Is TARGET2 Turbo Backing Valve Opened?", "Is BTL2 Turbo Backing Valve Opened?", "Is HPD Turbo Backing Valve Opened?", "Is M123 Backing at MID-VAC?", "Is OAP Backing at MID-VAC?", "Is TARGET1 Backing at MID-VAC?", "Is TARGET2 Backing at MID-VAC?", "Is BTL Backing at MID-VAC?", "Is BTL2 Backing at MID-VAC?", "Is HPD Backing at MID-VAC?", "Is M123 Turbo in Normal Operation", "Is COMP Turbo in Normal Operation", "Is OAP Turbo in Normal Operation", "Is BTL Turbo in Normal Operation", "Is TARGET1 Turbo in Normal Operation", "Is TARGET2 Turbo in Normal Operation", "Is BTL2 Turbo in Normal Operation", "Is HPD Turbo in Normal Operation", "Is M123 at MID-VAC?", "Is OAP at MID-VAC?", "Is COMP at MID-VAC?", "Is BTL at MID-VAC?", "Is TARGET at MID-VAC?", "Is BTL2 at MID-VAC?", "Is HPD at MID-VAC?"}
  T33 = typedef "command_typdef.ctl" = enum16{"No Action", "Set GPM Mode LB", "EXIT GPM Mode LB", "Set GPM Mode EC", "EXIT GPM Mode EC", "Set GVM mode LB", "Set GVM Mode EC", "Open LB Backing Valve", "Open EC Backing Valve", "Open EC Roughing Valve", "Open LB Roughing Valve", "Open M123 Roughing Valve", "Close M123 Roughing Valve", "Open Compressor Roughing Valve", "Close Compressor Roughing Valve", "Open BeamDump Roughing Valve", "Close BeamDump Roughing Valve", "Open OAP Roughing Valve", "Close OAP Roughing Valve", "Open BTL Roughing Valve", "Close BTL Roughing Valve", "Open Target Roughing Valve", "Close Target Roughing Valve", "Open BTL2 Roughing Valve", "Close BTL2 Roughing Valve", "Open HPD Roughing Valve", "Close HPD Roughing Valve", "LB Start Roughing Pump ", "EC Start Roughing Pump", "Open COMP Turbo Backing Valve", "Open M123 Turbo Backing Valve", "Open OAP Turbo Backing Valve", "Open HPBD Turbo Backing Valve", "Open BLT Turbo Backing Valve", "Open TARGET1 Turbo Backing Valve", "Open TARGET2 Turbo Backing Valve", "Open BLT2 Turbo Backing Valve", "Open HPD Turbo Backing Valve", "LB Start Turbo Backing Pump", "EC Start Turbo Backing Pump", "Start COMP Turbo Pump", "Start M123 Turbo Pump", "Start OAP Turbo Pump", "Start BTL Turbo Pump", "Start TARGET1 Turbo Pump", "Start TARGET2 Turbo Pump", "Start BTL2 Turbo Pump", "Start HPD Turbo Pump", "Open COMP Turbo Gate Valve", "Open M123 Turbo Gate Valve", "Open OAP Turbo Gate Valve", "Open BTL Turbo Gate Valve", "Open TARGET1 Turbo Gate Valve", "Open TARGET2 Turbo Gate Valve", "Open BTL2 Turbo Gate Valve", "Open HPD Turbo Gate Valve"}
  T34 = cluster{"boolarray1":cluster{bool, bool, bool, bool, bool, bool, bool, bool, bool, bool, bool, bool, bool, bool, bool, bool}, "boolarray2":cluster{bool, bool, bool, bool, bool, bool, bool, bool, bool, bool, bool, bool, bool, bool, bool, bool}, "boolarray3":cluster{bool, bool, bool, bool, bool, bool, bool, bool, bool, bool, bool, bool, bool, bool, bool, bool}, "boolarray4":cluster{bool, bool, bool, bool, bool, bool, bool, bool, bool, bool, bool, bool, bool, bool, bool, bool}}
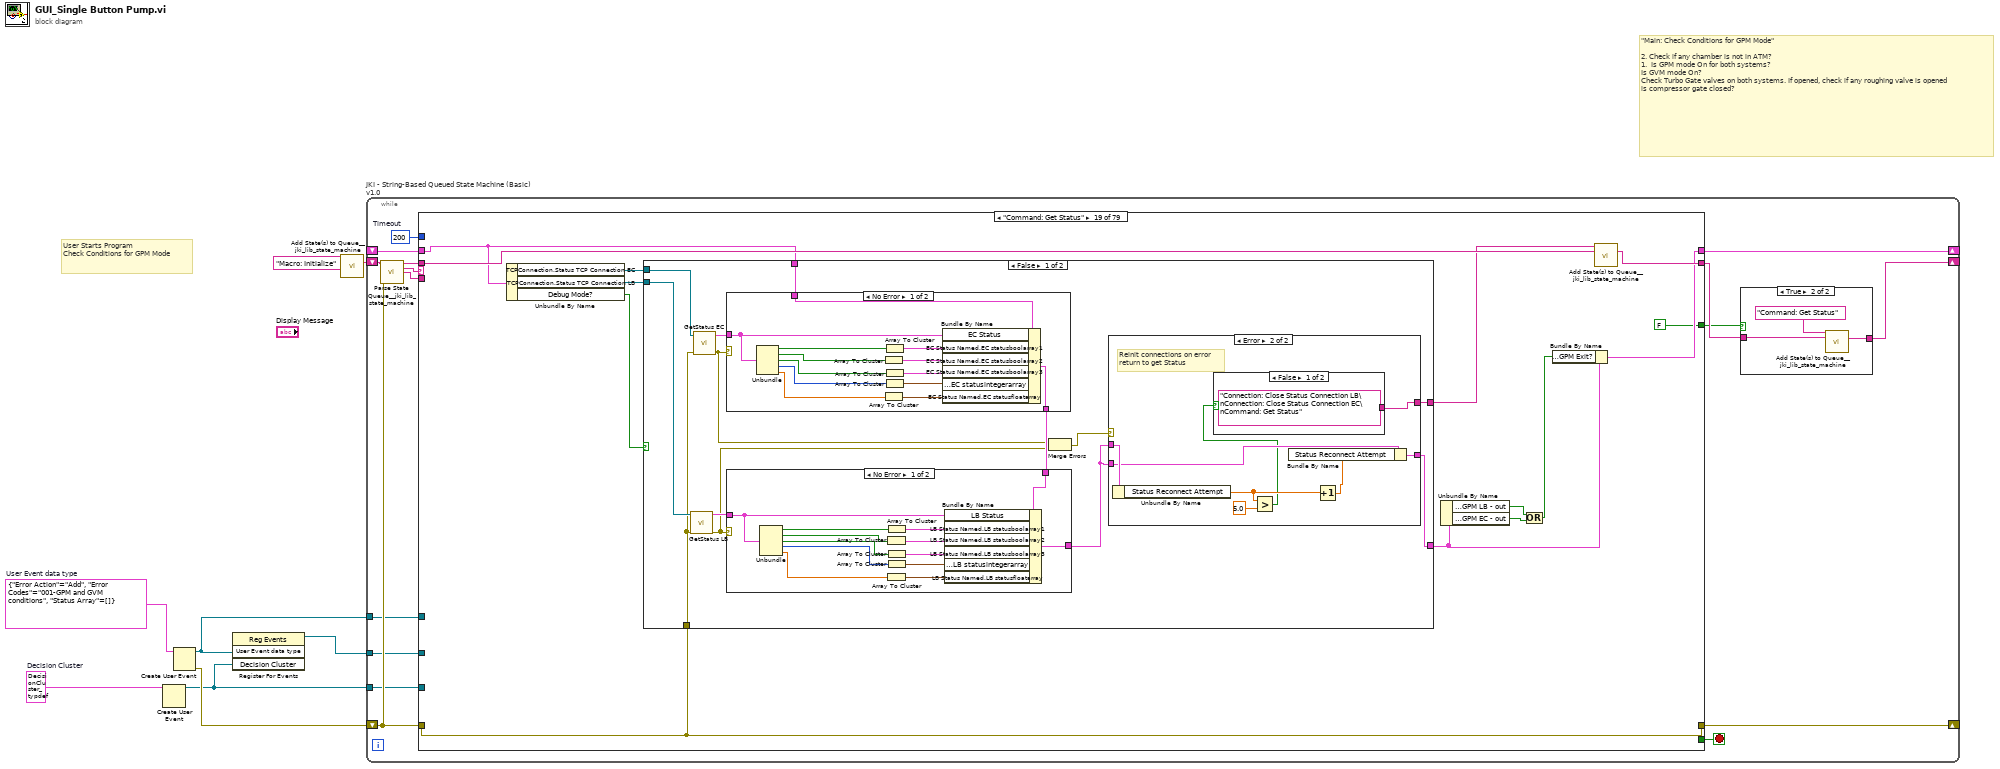
[diagram p0: block diagram]
diagram:
  w1 = T14 {"vi path"=path "Dummy.vi", "Message"=""}  # Decision Cluster
  w5 = T15 {"Error Action"=enum."Add", "Error Codes"=enum."001-GPM and GVM conditions", "Status Array"=[]}  # User Event data type
  # "\"Main: Check Conditions for GPM Mode\" \n\n2. Check if any chamber is not in ATM?\n1.  Is GPM mode On for both systems?\nIs GVM mode On?\nCheck Turbo Gate valves on both systems. If opened, check if any roughing valve is opened\nis compressor gate closed?"
  # "User Starts Program\nCheck Conditions for GPM Mode"
  n1 = Create User Event(user event datatype=w1) -> (user event=w2:refnum<user-event>)  [unwired: 1 in, 1 out]
  n2 = Create User Event(user event datatype=w5) -> (user event=w4:refnum<user-event>, error out=w3:errorcluster)  [unwired: 1 in]
  n3 = register-events(w4, w2) -> (reference out=w6:refnum<event-registration>)  [unwired: 2 in, 1 out]
  n4 = call <vilib>:"Add State(s) to Queue__jki_lib_state_machine.vi"("State(s) in (\"\")"="Macro: Initialize") -> ("States Out"=w8:string)  [unwired: 14 in]
  n5 = while "JKI - String-Based Queued State Machine (Basic) v1.0" {
    shift-right: [w18] -> _
    shift-left: _ -> [w17]
    shift-right: [w20] -> _
    shift-left: w3 -> [w15]
    shift-right: [w10] -> _
    shift-left: w8 -> [w21]
    tunnel: w6 -> [w14]
    tunnel: w4 -> [w13]
    tunnel: w2 -> [w12]
    stop <- w19 stop-if-true
    w16 = 200  # Timeout
    n6 = call <vilib>:"Parse State Queue__jki_lib_state_machine.vi"("State Queue"=w21, "Error In (no error)"=w15) -> ("Remaining States"=w23:string, "Current State"=w24:string, "Arguments"=w22:string)  [unwired: 11 in]
    n7 = case shown="\"Command: Get Status\"" w24 {
      selector: w24 -> [_ _ w126 _ _ _ _ _ _ _ _ _ _ _ _ _ _ _ _ _ _ _ _ _ _ _ _ _ _ _ _ _ _ _ _ _ _ _ _ _ _ _ _ _ _ _ _ _ _ _ _ _ _ _ _ _ _ _ _ _ _ _ _ _ _ _ _ _ _ _ _ _ _ _ _ _ _ _ _]
      tunnel: w23 -> [w37 w125 w130 w150 w156 w161 w165 w169 w183 w185 w197 w206 w217 w226 w237 w246 w260 w271 w277 w347 w351 w357 w368 w394 w401 w404 w417 w423 w433 w436 w526 w617 w708 w799 w890 w977 w1036 w1095 w1143 w1248 w1282 w1299 w1305 w1318 w1346 w1392 w1415 w1466 w1498 w1540 w1571 w1585 w1614 w1653 w1682 w1705 w1717 w1749 w1752 w1773 w1794 w1803 w1835 w1837 w1849 w1886 w1895 w1931 w1956 w1965 w2003 w2027 w2040 w2058 w2131 w2216 w2233 w2251 w2286]
      tunnel: w22 -> [_ _ _ _ _ _ _ _ _ _ _ _ _ _ _ _ _ _ _ _ _ w352 w362 _ _ _ _ _ _ w437 w527 w618 w709 w800 w891 w978 _ _ w1135 _ _ _ _ _ _ _ _ _ _ _ _ _ w1596 w1639 w1673 _ _ _ _ _ _ _ _ _ _ _ _ _ _ _ _ _ _ w2050 w2114 _ _ _ _]
      tunnel: w17 -> [w35 w122 w128 w141 w153 w159 w162 _ w179 w186 w192 w204 w212 w224 w232 w244 w255 w269 w276 w344 w349 w355 w364 w391 w398 w406 w419 w420 w432 w441 w531 w622 w713 w804 w894 w976 w1025 w1071 w1127 w1231 w1281 w1298 w1306 w1311 w1345 w1393 w1398 w1449 w1497 w1522 w1572 w1578 w1600 w1641 w1667 w1706 w1708 w1732 w1751 w1754 w1775 w1796 w1816 w1838 w1842 w1865 w1888 w1914 w1934 w1958 w1983 w2005 w2033 w2049 w2116 w2204 w2221 w2237 w2283]
      tunnel: [w34 w123 w132 w147 errorcluster {"status"=FALSE, "code"=0, "source"=""} ("error out") w158 w163 w167 w180 w184 w189 w201 w209 w221 w229 w241 w252 w266 w274 w345 w348 w353 w365 w392 w399 w403 w416 w421 w425 w444 w534 w625 w716 w807 w897 w983 w1030 w1088 w1136 w1243 w1280 w1290 w1304 w1312 w1359 w1391 w1408 w1459 w1500 w1533 w1570 w1583 w1611 w1642 w1675 w1704 w1713 w1741 w1750 w1765 w1786 w1798 w1827 w1836 w1844 w1879 w1890 w1930 w1949 w1960 w1996 w2020 w2038 w2054 w2124 w2205 w2223 w2244 w2284] -> w20
      tunnel: w15 -> [w33 w123 w131 w147 w152 w158 w163 w167 w175 w184 w189 w202 w209 w222 w229 w242 w252 w267 w274 w345 w348 w354 w366 w392 w399 w403 w416 w421 w425 w446 w536 w627 w718 w809 w899 w985 w1033 w1091 w1141 w1245 w1280 w1290 w1304 w1315 w1354 w1391 w1413 w1464 w1503 w1538 w1570 w1583 w1610 w1646 w1680 w1704 w1715 w1746 w1750 w1770 w1791 w1801 w1832 w1836 w1847 w1884 w1893 w1930 w1954 w1963 w2001 w2025 w2038 w2056 w2129 w2210 w2227 w2249 w2284]
      tunnel: [w36 w124 w129 w149 w155 w160 w164 w168 w182 w185 w196 w205 w216 w225 w236 w245 w259 w270 w278 w346 w350 w356 w367 w393 w400 w405 w418 w422 w434 w447 w537 w628 w719 w810 w900 w986 w1035 w1094 w1142 w1247 w1285 w1301 w1305 w1317 w1361 w1392 w1414 w1465 w1504 w1539 w1571 w1584 w1613 w1652 w1681 w1705 w1716 w1748 w1752 w1772 w1793 w1802 w1834 w1837 w1848 w1885 w1894 w1932 w1955 w1964 w2002 w2026 w2039 w2057 w2130 w2215 w2232 w2250 w2285] -> w11
      tunnel: [_ _ _ _ _ TRUE _ _ _ _ _ _ _ _ _ _ _ _ _ _ _ _ _ _ _ _ _ _ _ _ _ _ _ _ _ _ _ _ _ _ _ _ _ _ _ _ _ _ _ _ _ _ _ _ _ _ _ _ _ _ _ _ _ _ _ _ _ _ _ _ _ _ _ _ _ _ _ _ _] -> w19
